vi "Get_TempHum_CalValues.vi"() -> (0 "Inside temp.":sgl, 1 "Outside temp.":sgl, 3 "Offset outside hum.":i32, 4 "Offset inside hum.":i32, 5 "Inside hum.":sgl, 6 "Outside hum.":sgl, 7 "TempHum read?":bool, 8 "Offset outside temp.":sgl, 9 "Offset inside temp.":sgl)   [LabVIEW 2013]
uses:
  VantagePro.dll
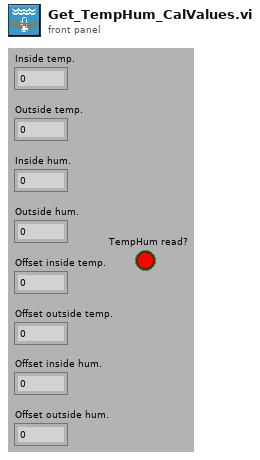
[diagram p1: front panel]
types:
  T1 = cluster{"In Temp":sgl, "Out Temp":sgl, "In Hum":u8, "Out Hum":u8, "Dum":i8, "Dum":i8, "Off In Temp":sgl, "Off Out Temp":sgl, "Off In Hum":i8, "Off Out Hum":i8}
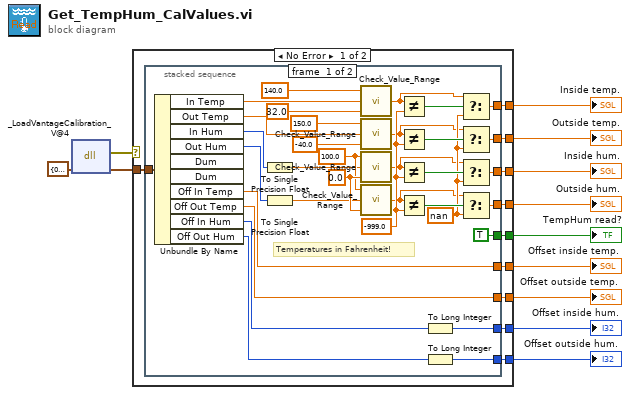
[diagram p0: block diagram]
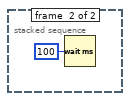
[diagram p2: hidden frame]
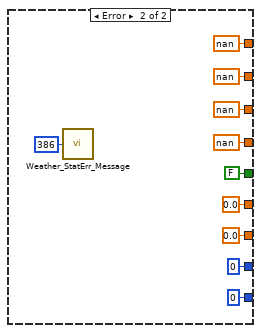
[diagram p3: hidden frame]
diagram:
  n1 = dll-call lib="C:/Users/vaneijk/Documents/LabView Projects 13/HiSPARC Weather Station/Develop/VantagePro.dll" fn="_LoadVantageCalibration_V@4" label="Temp&hum data"("calibration"=T1 {"In Temp"=0.0, "Out Temp"=0.0, "In Hum"=0, "Out Hum"=0, "Dum"=0, "Dum"=0, "Off In Temp"=0.0, "Off Out Temp"=0.0, "Off In Hum"=0, "Off Out Hum"=0}) -> (error out=w1:errorcluster, "calibration"=w2:T1)  [unwired: 4 in, 1 out]
  n2 = case shown="No Error" w1 {
    tunnel: w2 -> [w22 _]
    tunnel: [w21 sgl nan ("Data_input")] -> w12
    tunnel: [w20 sgl nan ("Data_input")] -> w11
    tunnel: [w19 sgl nan ("Data_input")] -> w10
    tunnel: [w18 sgl nan ("Data_input")] -> w9
    tunnel: [w17 0] -> w8
    tunnel: [w16 0] -> w7
    tunnel: [w15 sgl 0.0 ("Data_input")] -> w6
    tunnel: [w14 sgl 0.0 ("Data_input")] -> w5
    tunnel: [w13 FALSE] -> w4
    frame No Error {
      n3 = stacked-sequence {
        tunnel: w22 -> [w56 _]
        tunnel: [w39 _] -> w21
        tunnel: [w38 _] -> w20
        tunnel: [w37 _] -> w19
        tunnel: [w36 _] -> w18
        tunnel: [w35 _] -> w17
        tunnel: [w34 _] -> w16
        tunnel: [w24 _] -> w15
        tunnel: [w23 _] -> w14
        tunnel: [TRUE _] -> w13
        frame #0 {
          w40 = sgl nan ("Data_input")
          w45 = sgl -999.0 ("Min")
          w53 = sgl 0.0 ("Min")
          w52 = sgl 100.0 ("Max")
          # "Temperatures in Fahrenheit!"
          n4 = Unbundle By Name(w56) -> ("In Temp"=w31:sgl, "Out Temp"=w32:sgl, "In Hum"=w49:u8, "Out Hum"=w48:u8, "Off In Temp"=w24:sgl, "Off Out Temp"=w23:sgl, "Off In Hum"=w55:i8, "Off Out Hum"=w54:i8)  [unwired: 2 out]
          n5 = To Single Precision Float(number=w49) -> (single precision float=w47:sgl)
          n6 = To Single Precision Float(number=w48) -> (single precision float=w46:sgl)
          n7 = call "Check_Value_Range.vi"("Min"=sgl 32.0, "Data in"=w31, "Max"=sgl 140.0) -> ("Data out"=w28:sgl)
          n8 = call "Check_Value_Range.vi"("Min"=sgl -40.0, "Data in"=w32, "Max"=sgl 150.0) -> ("Data out"=w27:sgl)
          n9 = call "Check_Value_Range.vi"("Min"=w53, "Data in"=w47, "Max"=w52) -> ("Data out"=w26:sgl)
          n10 = call "Check_Value_Range.vi"("Min"=w53, "Data in"=w46, "Max"=w52) -> ("Data out"=w25:sgl)
          n11 = Not Equal?(x=w28, y=w45) -> (x != y?=w44:bool)
          n12 = Not Equal?(x=w27, y=w45) -> (x != y?=w42:bool)
          n13 = Not Equal?(x=w26, y=w45) -> (x != y?=w41:bool)
          n14 = Not Equal?(x=w25, y=w45) -> (x != y?=w43:bool)
          n15 = To Long Integer(number=w55) -> (32bit integer=w35:i32)
          n16 = To Long Integer(number=w54) -> (32bit integer=w34:i32)
          n17 = Select(t=w28, s=w44, f=w40) -> (s? t:f=w39:sgl)
          n18 = Select(t=w27, s=w42, f=w40) -> (s? t:f=w38:sgl)
          n19 = Select(t=w26, s=w41, f=w40) -> (s? t:f=w37:sgl)
          n20 = Select(t=w25, s=w43, f=w40) -> (s? t:f=w36:sgl)
        }
        frame #1 {
          n21 = Wait (ms)(milliseconds to wait=u32 100 ("millisecond multiple")) -> ()  [unwired: 1 out]
        }
      }
    }
    frame Error {
      n22 = call "Weather_StatErr_Message.vi"("Message number"=386) -> ()  [unwired: 1 out]
    }
  }
  "Offset outside hum." <- w7
  "Offset inside hum." <- w8
  "Offset outside temp." <- w5
  "Offset inside temp." <- w6
  "Outside hum." <- w9
  "Inside hum." <- w10
  "Outside temp." <- w11
  "Inside temp." <- w12
  "TempHum read?" <- w4
